vi "[Property] Fahrenheit Mode Write.vi"(4 "error in (no error)":errorcluster, 5 "Value":bool, 6 "Container State":T2, 7 "Display State In":T1) -> (0 "error out":errorcluster, 3 "Display State Out":T1)   [LabVIEW 2012, in "Simple Dual Mode Thermometer XControl.xctl"]
doc: "This VI handles the Fahrenheit? Write property as part of the Simple Dual Mode Thermometer XControl."
uses:
  Simple Dual Mode Thermometer XControl.xctl
  <vilib>/_xctls/Container State.ctl
  Simple Dual Mode Thermometer State.ctl
  <vilib>/_xctls/XControlSupport.lvlib
panel:
  # "See block diagram"
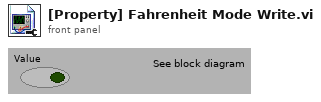
[diagram p1: front panel]
types:
  T1 = typedef "Simple Dual Mode Thermometer XControl.xctl/Simple Dual Mode Thermometer State.ctl" = cluster{"Fahrenheit":bool}
  T2 = typedef "XControlSupport.lvlib/Container State.ctl" = cluster{"Indicator?":bool, "Run Mode?":bool, " Refnum":refnum<vi>}
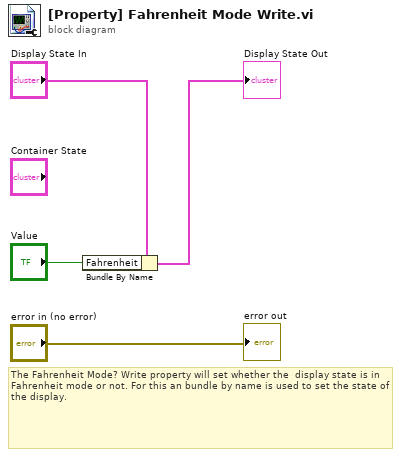
[diagram p0: block diagram]
diagram:
  # "The Fahrenheit Mode? Write property will set whether the  display state is in Fahrenheit mode or not. For this an bundle by name is used to set the state of the display."
  n1 = Bundle By Name(cluster="Display State In", "Fahrenheit"="Value") -> (→"Display State Out":T1)
  "error out" <- "error in (no error)"
